vi "CheckMenuPan.vi"(8 "error in (no error)":errorcluster caption="entrée d'erreur (pas d'erreur)", 9 "Function":string, 10 "LoadedFuncArr":string[](array[string]), 11 "LoadedInst":refnum<class "BaseDevice.lvclass">[](array[class])) -> (0 "error out":errorcluster caption="sortie d'erreur", 1 "PanelName":string="ClassPanel", 2 "MenuPanInstrInd":i32, 3 "LoadedInst Out":refnum<class "BaseDevice.lvclass">[](array[class]), 5 "OperCanceled":bool)   [LabVIEW 2019, in "BaseDevice.lvclass"]
uses:
  BaseDevice.lvclass
  BaseDevice.lvclass/BaseDevice.ctl
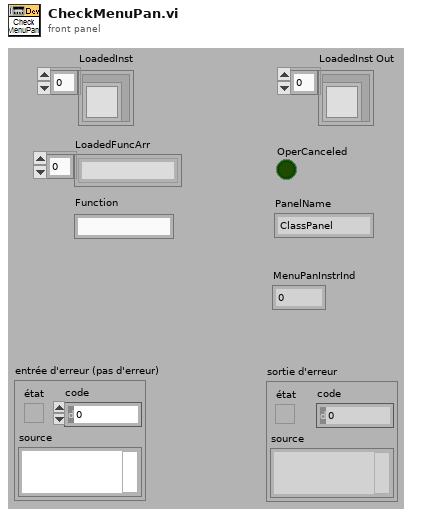
[diagram p1: front panel]
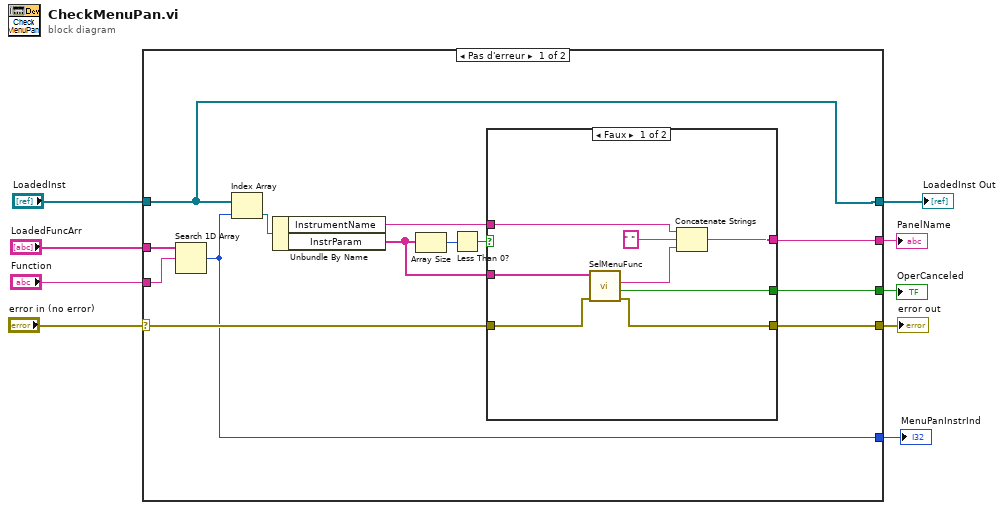
[diagram p0: block diagram]
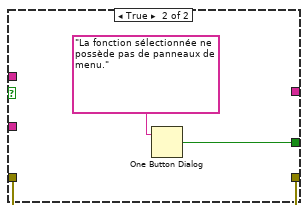
[diagram p2: hidden frame]
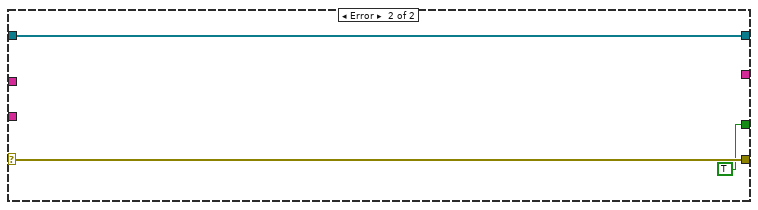
[diagram p3: hidden frame]
diagram:
  n1 = case shown="Pas d'erreur" "error in (no error)" {
    selector: "error in (no error)" -> [w18 w36]
    tunnel: [w17 w36] -> w8
    tunnel: "LoadedInst" -> [w12 w35]
    tunnel: "LoadedFuncArr" -> [w22 _]
    tunnel: "Function" -> [w19 _]
    tunnel: [w21 TRUE ("Canceled")] -> w4
    tunnel: [w20 _] -> w3
    tunnel: [w12 w35] -> w2
    tunnel: [w11 _] -> w1
    frame No Error {
      n2 = Search 1D Array(1D array=w22, element=w19) -> (index of element=w11:i32)  [unwired: 1 in]
      n3 = Index Array(array=w12, index=w11) -> (element=w13:refnum<class "BaseDevice.lvclass">)
      n4 = Unbundle By Name(w13) -> ("InstrumentName"=w10:string, "InstrParam"=w14:string[])
      n5 = Array Size(array=w14) -> (size(s)=w15:i32)
      n6 = Less Than 0?(x=w15) -> (x < 0?=w16:bool)
      n7 = case shown="Faux" w16 {
        tunnel: [w29 w31] -> w21
        tunnel: [w28 _] -> w20
        tunnel: w14 -> [w30 _]
        tunnel: w18 -> [w26 w32]
        tunnel: [w25 w32] -> w17
        tunnel: w10 -> [w23 _]
        frame False {
          n8 = call "SelMenuFunc.vi"("error in (no error)"=w26, "AvailFunc"=w30) -> ("error out"=w25:errorcluster, "Canceled"=w29:bool, "Selected Panel"=w24:string)  [unwired: 6 in, 1 out]
          n9 = Concatenate Strings(w23, " " ("chaîne"), w24) -> (w28:string)
        }
        frame True {
          n10 = One Button Dialog(message="La fonction sélectionnée ne possède pas de panneaux de menu.") -> (true=w31:bool)  [unwired: 1 in]
        }
      }
    }
    frame Error {
    }
  }
  "error out" <- w8
  "OperCanceled" <- w4
  "PanelName" <- w3
  "LoadedInst Out" <- w2
  "MenuPanInstrInd" <- w1
